vi "LFA_AcquireAltSPEMethod.vi"(8 "error in (no error)":errorcluster, 10 "Delete File?":bool, 11 "LightField Automation in":refnum<class "LightField Automation.lvclass">) -> (0 "error out":errorcluster, 2 "Data":T1(array[cluster]), 3 "LightField Automation out":refnum<class "LightField Automation.lvclass">)   [LabVIEW 2013, in "LightField Automation.lvclass"]
uses:
  LightField Automation.lvclass
  LightField Automation.lvclass/LightField Automation.ctl
  C:/Program Files/Princeton Instruments/LightField/AddInViews/PrincetonInstruments.LightFieldViewV3.dll
  Program Files/Princeton Instruments/LightField/AddInViews/PrincetonInstruments.LightFieldViewV3.dll
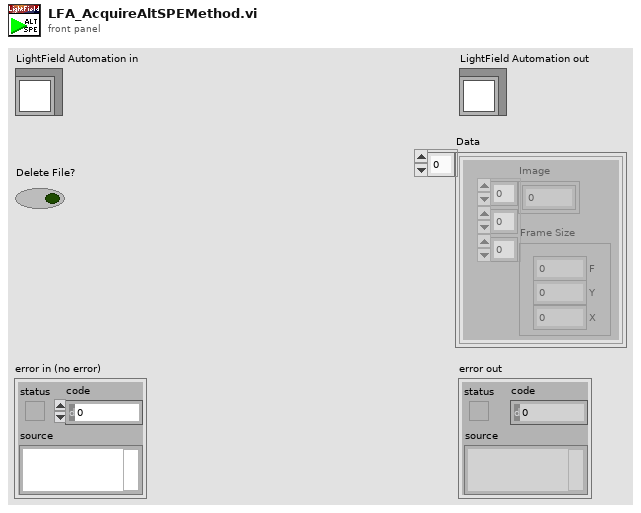
[diagram p1: front panel]
types:
  T1 = cluster{"Image":dbl[][][], "Frame Size":cluster{"F":i32, "Y":i32, "X":i32}}[]
  T2 = cluster{"ROI Height":i32[], "ROI Width":i32[], "ROI Stride":i32[], "ROI Size":i64[]}
  T3 = cluster{"Pixel Format":string, "Number of Frames":i32, "Frame Size":i32, "Frame Stride":i64}
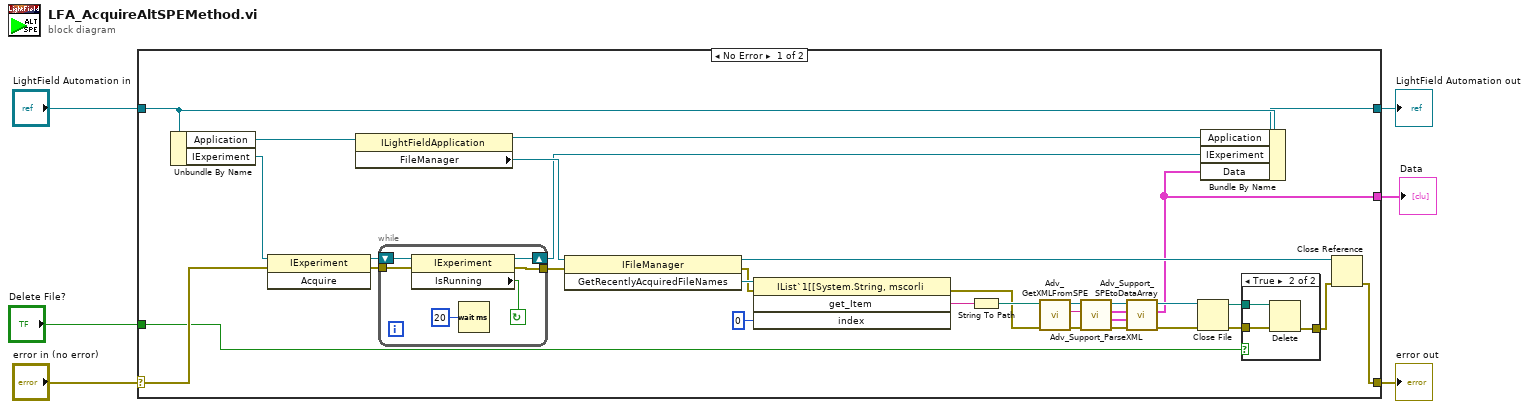
[diagram p0: block diagram]
diagram:
  n1 = case shown="No Error" "error in (no error)" {
    selector: "error in (no error)" -> [w39 w51]
    tunnel: [w29 w51] -> w5
    tunnel: [w14 w50] -> w3
    tunnel: "LightField Automation in" -> [w15 w50]
    tunnel: [w13 _] -> w2
    tunnel: "Delete File?" -> [w9 _]
    frame No Error {
      n2 = Unbundle By Name(w15) -> ("Application"=w35:refnum<k24>, "IExperiment"=w36:refnum<k24>)
      n3 = invoke class="IExperiment" method="Acquire"(reference=w36, error in=w39) -> (reference out=w37:refnum<k24>, error out=w38:errorcluster)  [unwired: 1 in, 1 out]
      n4 = property class="ILightFieldApplication"(reference=w35) -> (reference out=w8:refnum<k24>, "FileManager"=w34:refnum<k24>)  [unwired: 1 in, 1 out]
      n5 = while {
        tunnel: w38 -> [w47]
        tunnel: [w46] -> w33
        shift-right: [w44] -> w7
        shift-left: w37 -> [w45]
        stop <- w49 continue-if-true
        n6 = property class="IExperiment"(reference=w45, error in=w47) -> (reference out=w44:refnum<k24>, error out=w46:errorcluster, "IsRunning"=w49:bool)
        n7 = Wait (ms)(milliseconds to wait=u32 20) -> ()  [unwired: 1 out]
      }
      n8 = invoke class="IFileManager" method="GetRecentlyAcquiredFileNames"(reference=w34, error in=w33) -> (reference out=w28:refnum<k24>, error out=w31:errorcluster, "GetRecentlyAcquiredFileNames"=w32:refnum<k24>)  [unwired: 1 in]
      n9 = invoke class="IList`1[[System.String, mscorli" method="get_Item"(reference=w32, error in=w31, "index"=0) -> (error out=w25:errorcluster, "get_Item"=w27:string)  [unwired: 1 in, 2 out]
      n10 = String To Path(string=w27) -> (path=w26:path)
      n11 = call "Adv_GetXMLFromSPE.vi"("error in (no error)"=w25, "Path In"=w26) -> ("error out"=w22:errorcluster, "XML"=w23:string, "SPE Refnum"=w24:refnum<file>)  [unwired: 7 in]
      n12 = call "Adv_Support_ParseXML.vi"("error in (no error)"=w22, "XML"=w23, "SPE Refnum"=w24) -> ("error out"=w18:errorcluster, "ROI Info"=w19:T2, "Frame Info"=w20:T3, "SPE Refnum"=w21:refnum<file>)  [unwired: 5 in]
      n13 = call "Adv_Support_SPEtoDataArray.vi"("error in (no error)"=w18, "ROI Info"=w19, "Frame Info"=w20, "SPE Refnum"=w21) -> ("error out"=w17:errorcluster, "Data"=w13:T1, "SPE Refnum 2"=w16:refnum<file>)  [unwired: 5 in]
      n14 = Close File(refnum=w16, error in=w17) -> (path=w11:path, error out=w12:errorcluster)
      n15 = Bundle By Name(cluster=w15, "Application"=w8, "IExperiment"=w7, "Data"=w13) -> (w14:refnum<class "LightField Automation.lvclass">)
      n16 = case shown="True" w9 {
        tunnel: w12 -> [w40 w43]
        tunnel: w11 -> [_ w42]
        tunnel: [w40 w41] -> w10
        frame False {
        }
        frame True {
          n17 = Delete(path (use dialog)=w42, error in=w43) -> (error out=w41:errorcluster)  [unwired: 3 in, 2 out]
        }
      }
      n18 = Close Reference(reference=w28, error in (no error)=w10) -> (error out=w29:errorcluster)
    }
    frame Error {
    }
  }
  "error out" <- w5
  "LightField Automation out" <- w3
  "Data" <- w2
